vi "radar_data_cube_plotter.vi"(0 "Radar cube":string, 1 "FFT size":i32=512, 2 "error in":errorcluster) -> (3 "#samples per frame (complex)":i32=339200, 4 "Fast Channel FFT":cluster{sgl, sgl, sgl[]}(graph), 5 "Sweep Response":cluster{sgl, sgl, sgl[]}(graph), 6 "error out":errorcluster)   [LabVIEW 2019, in "Lib_Simx.lvlib"]
doc: "Use to calculate the Fast Fourier transform (FFT) of the radar cube."
uses:
  <vilib>/Analysis/2dsp.llb/Complex FFT.vi
  Lib_Simx.lvlib
  <vilib>/Analysis/NI_AALPro.lvlib
panel:
  in  "element number":i32
  in  "sweep number":i32
  in  "#elements":i32=8
  in  "#sweeps":i32=32
  in  "#samples per sweep":i32=345
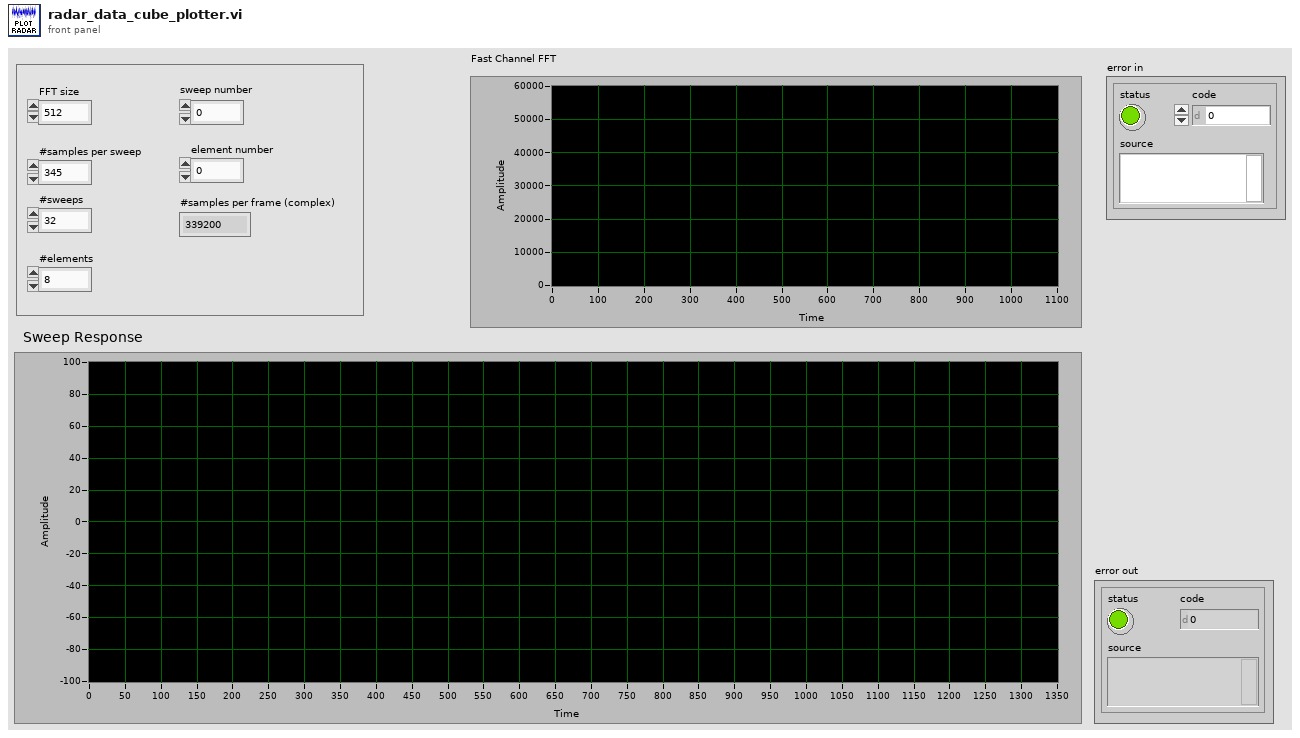
[diagram p1: front panel]
types:
  T1 = enum16{"big-endian, network order", "native, host order", "little-endian"}
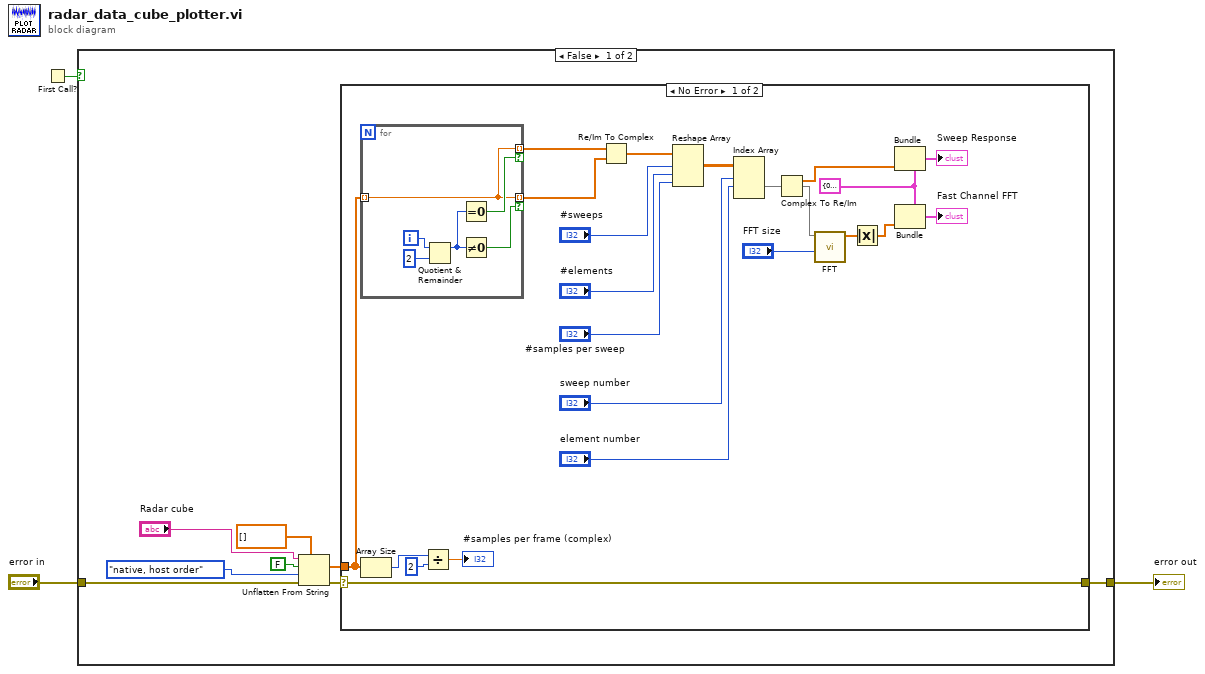
[diagram p0: block diagram]
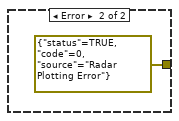
[diagram p2: hidden frame]
diagram:
  n1 = First Call?() -> (First Call?: T/F=w3:bool)
  n2 = case shown="False" w3 {
    tunnel: "error in" -> [w5 w41]
    tunnel: [w4 w41] -> w1
    frame False {
      n3 = Unflatten From String(type=sgl[] [], binary string="Radar cube", data includes array or string size? (T)=FALSE, byte order (0:big-endian, network order)=T1."native, host order" ("byte order (0:big-endian, network order) 2"), error in (no error)=w5) -> (value=w6:sgl[], error out=w8:errorcluster)  [unwired: 1 out]
      n4 = case shown="No Error" w8 {
        selector: w8 -> [w18 _]
        tunnel: w6 -> [w14 _]
        tunnel: [w18 errorcluster {"status"=TRUE, "code"=0, "source"="Radar Plotting Error"} ("error in (no error)")] -> w4
        frame No Error {
          w27 = cluster{sgl, sgl, sgl[]} {0.0, 0.0, []}
          n5 = for {
            tunnel: w14 -> [w35] mode=indexing
            tunnel: [w35] -> w13 mode=indexing if=w37
            tunnel: [w35] -> w12 mode=indexing if=w34
            i -> [w39]
            n6 = Quotient & Remainder(x=w39, y=2) -> (x-y*floor(x/y)=w36:i32)  [unwired: 1 out]
            n7 = Equal To 0?(x=w36) -> (x = 0?=w37:bool)
            n8 = Not Equal To 0?(x=w36) -> (x != 0?=w34:bool)
          }
          n9 = Array Size(array=w14) -> (size(s)=w31:i32)
          n10 = Divide(x=w31, y=2) -> (x/y=→"#samples per frame (complex)":dbl)
          n11 = Re/Im To Complex(1:w12, 2:w13) -> (0:w23:csg[])
          n12 = Reshape Array(w23, "#sweeps", "#elements", "#samples per sweep") -> (w21:csg[][][])
          n13 = Index Array(array=w21, index (dim 0)="sweep number", index (dim 1)="element number") -> (element=w15:csg[])  [unwired: 1 in]
          n14 = Complex To Re/Im(x + iy=w15) -> (x=w33:sgl[])  [unwired: 1 out]
          n15 = call-poly <vilib>:"FFT.vi"("FFT size"="FFT size", "X"=w15) -> ("FFT {X}"=w32:cdb[])  [unwired: 8 in, 1 out]
          n16 = Absolute Value(x=w32) -> (abs(x)=w26:dbl[])
          n17 = Bundle(cluster=w27, w33) -> (→"Sweep Response":cluster{sgl, sgl, sgl[]})  [unwired: 2 in]
          n18 = Bundle(cluster=w27, w26) -> (→"Fast Channel FFT":cluster{sgl, sgl, sgl[]})  [unwired: 2 in]
        }
        frame Error {
        }
      }
    }
    frame True {
    }
  }
  "error out" <- w1
